vi "FaulhaberV3_Standalone.vi"() -> ()   [LabVIEW 2011]
panel:
  in  "1:x":i32(slide)=700 scale=-250000.0..250000.0
  in  "Tab Control":enum32{"command", "Script"}(tab)
  in  "commands":string[](array[string])=["Controlword?", "Modes of operation?", "Statusword?", "Position Actual Value?", "Controlword=0xF", "Modes of operation=1", "TargetPosition=-12345", "Controlword=0xF", "Controlword=0x1F", "Homing Method=37", "Modes of operation=6", "HomeOffset=23456", "Profile velocity?", "Profile velocity=1000", "Profile acceleration?", "Profile deceleration?", "Torque control parameters_Gain Kpi?", "Device data_Device nominal current?", "Device temperature_Winding temperature?", "Actual values_Motor current Id actual value?", "Current actual value?", "Motion profile type?", "Device Status?", "", "", "", "", ""]
  in  "Run":bool[](array[boolean])=[FALSE, FALSE, FALSE, FALSE, FALSE, FALSE, FALSE, FALSE, FALSE, FALSE, FALSE, FALSE, FALSE, FALSE, FALSE, FALSE, FALSE, FALSE, FALSE, FALSE, FALSE, FALSE, FALSE]
  out "return name":string="5000\r\n"
  out "return":i32
  out "Binary":bool[](array[boolean])
  out "Cluster 2":T1={"command"="goto abs", "Numeric"=0.0, "wait ms"=1000, "expected ssi"=235298.717399, "String"="go to low"}
  in  "start":bool
  out "Waveform Chart":dbl(graph)=2342.2826010000135
  in  "Timeout ms":i32=-1
  in  "Export ascii":bool
  in  "read ascii":bool
  in  "Next#":i32=259
  in  "List":T2(array[cluster])=[{"command"="LA", "Numeric"=30000.0, "wait ms"=10, "expected ssi"=0.0, "String"=""}, {"command"="M", "Numeric"=nan, "wait ms"=1000, "expected ssi"=0.0, "String"=""}, {"command"="LA", "Numeric"=0.0, "wait ms"=10, "expected ssi"=0.0, "String"=""}, {"command"="M", "Numeric"=nan, "wait ms"=1000, "expected ssi"=0.0, "String"=""}, {"command"="LA", "Numeric"=-30000.0, "wait ms"=10, "expected ssi"=0.0, "String"=""}, {"command"="M", "Numeric"=nan, "wait ms"=1000, "expected ssi"=0.0, "String"=""}, {"command"="LA", "Numeric"=0.0, "wait ms"=10, "expected ssi"=0.0, "String"=""}, {"command"="M", "Numeric"=nan, "wait ms"=1000, "expected ssi"=0.0, "String"=""}]
  in  "allowed ssi error":dbl=2000.0
  out "ssi in range":bool
  out "connect OK":bool
  out "error out":errorcluster
  in  "stop":bool
  in  "Axis # (nur1)":i16=1
  in  "Port, enter before start":refnum<visa-resource-name>="COM10"
  # "christianb:com10,D:com8"
  # "60000=10mm"
  # "closes comport\notherwise use STOP"
  # "Status ro\n0  ready on\n1 On\n2 Enabled\n3 Fault\n4 volt enabled\n5 quickstop\n6 on disabled\n7 Warning\n8 \n9 \n10 reached\n11 internal limit\n12  new point acept\n 13 follow error"
  # "Control\n0 on\n1 enable\n2 quick stop\n3 enable\n4 take set\n5 take immediately\n6 is relative\n7 faultreset\n8 halt\n9 no stop \n10 reached\n11\n12 point Acq"
  # "Einschalten\nControlword=0xF   Bit0,1,2,3, vorher 0x6?\nModes of operation=1 (PP)\n\nFahren\nTargetPosition=1234\nControlword=0xF könnte auch vorher sein\nControlword=0x1F  bit4 setzen, steigend=go, oder 3F sofort\n\nHoming method=37\nModes of operation=6 (Homing)\nHomeOffset=2345\nControlword=0x1F  bit 4 setzen\n?"
  # "software limits: \nPosition range limit_Min position range limit\nPosition range limit_Max position range limit\nSoftware position limit_Min position limit\nGNL, GPL\nSet LL<0, LL>0\nTEM Temperatur\nLPC 500  (mA)"
  # "Abfragen:\nPosition Actual Value?\nGAC\nGSP\nGRC  aktuelleer Strom\nG..."
  # "Parameter\nAC 5000\nDEC 5000\nSP 3000 (RPM=25mm/s)"
  # "-1 = stop\n>=0 restart"
  # "NaN expectet will not be checked"
  # "verlorener schritt=256*4 ysteps\nhalber ~200ssi (400 z)"
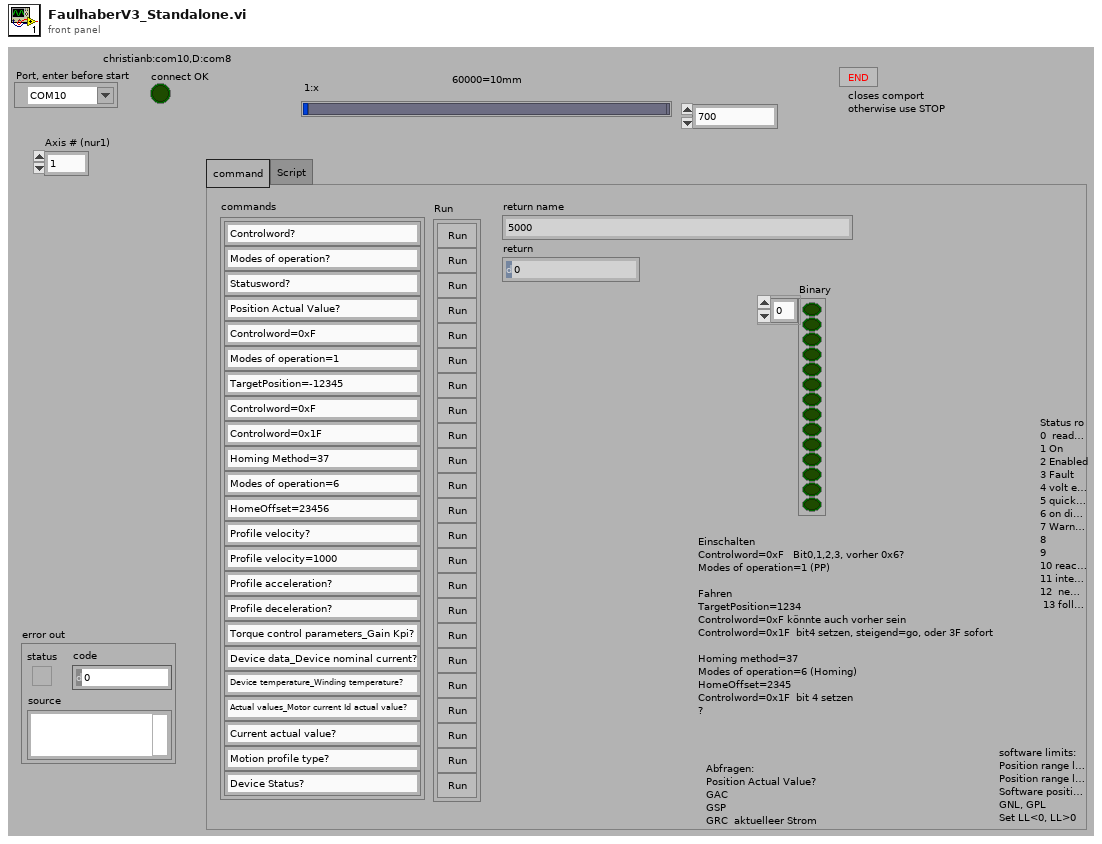
[diagram p1: front panel]
types:
  T1 = cluster{"command":string, "Numeric":dbl, "wait ms":i32, "expected ssi":dbl, "String":string}
  T2 = cluster{"command":string, "Numeric":dbl, "wait ms":i32, "expected ssi":dbl, "String":string}[]
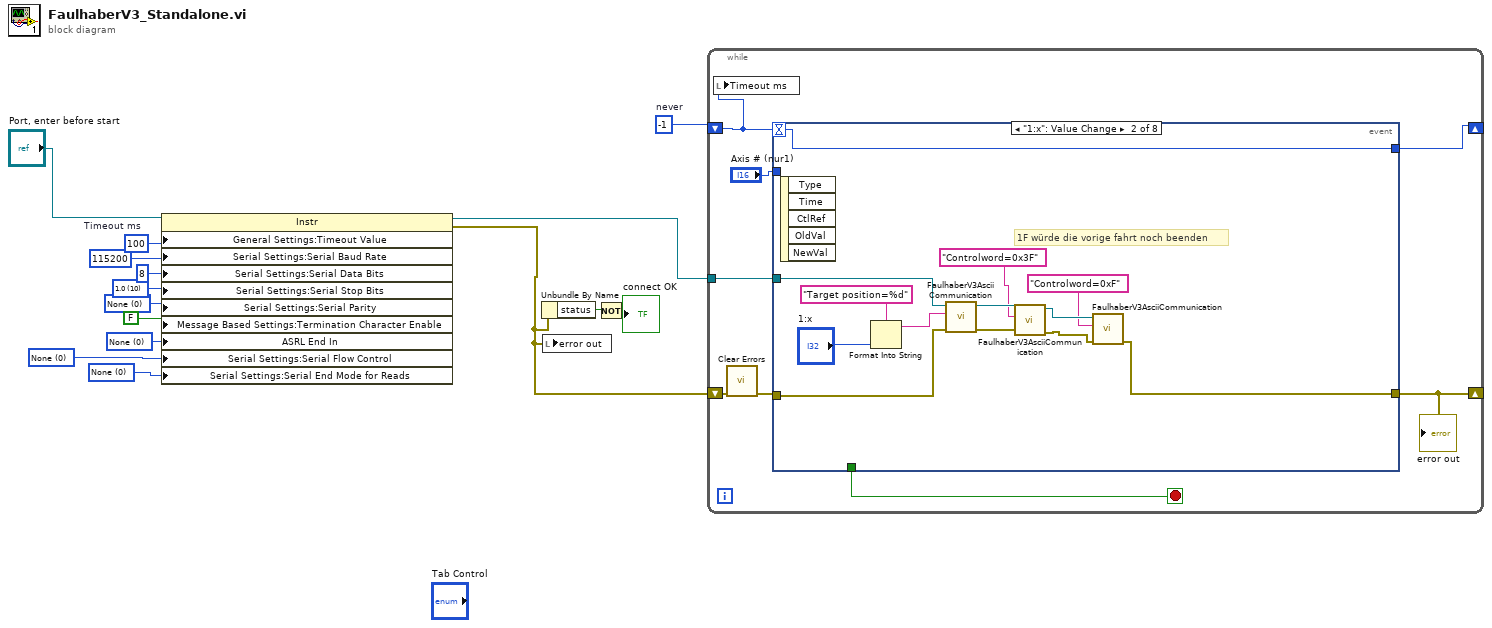
[diagram p0: block diagram]
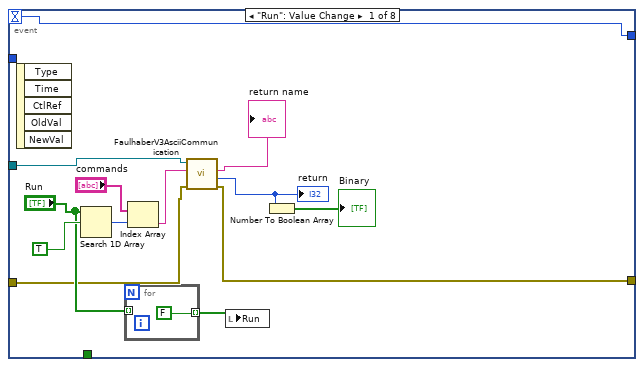
[diagram p2: hidden frame]
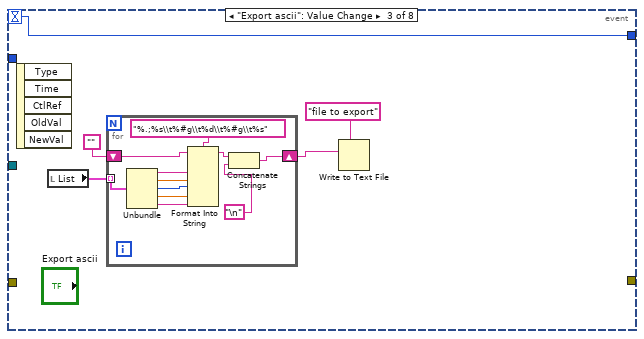
[diagram p3: hidden frame]
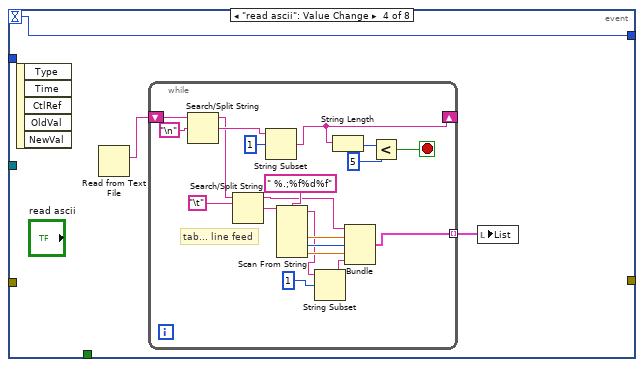
[diagram p4: hidden frame]
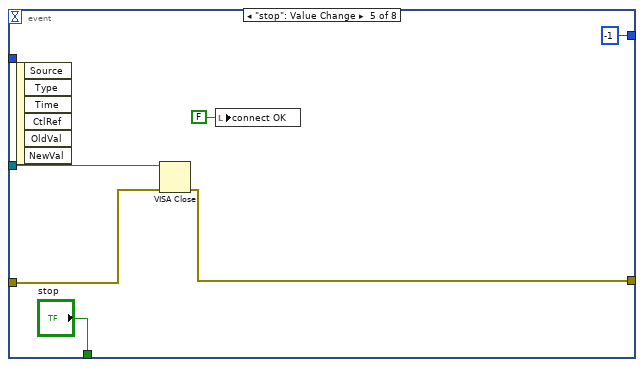
[diagram p5: hidden frame]
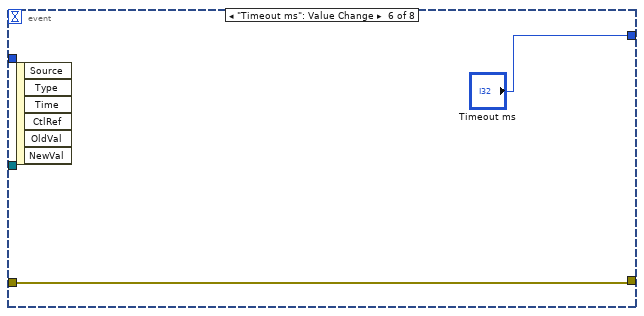
[diagram p6: hidden frame]
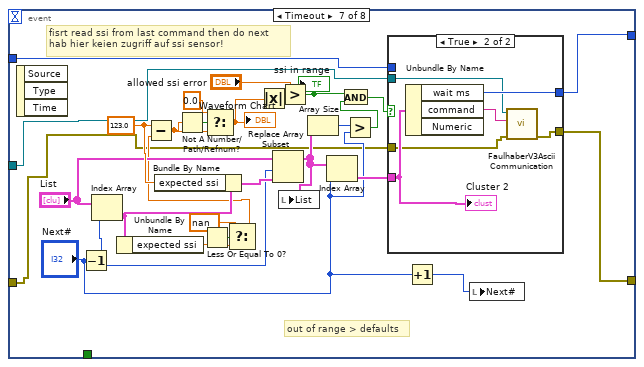
[diagram p7: hidden frame]
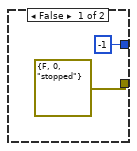
[diagram p8: hidden frame]
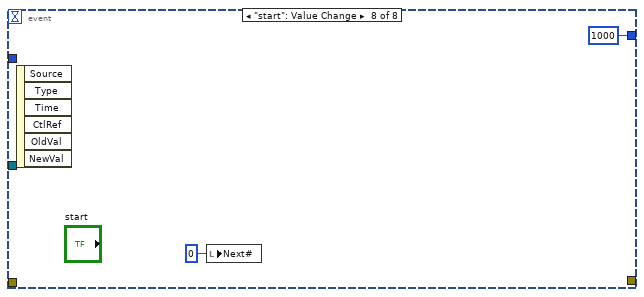
[diagram p9: hidden frame]
diagram:
  w2 = u16 0 items=["None", "Last Bit", "TermChar"] ("Serial Settings:End Mode for Reads")
  w7 = u32 100  # Timeout ms
  w9 = u16 10 items=["1.0"=10, "1.5"=15, "2.0"=20] ("Serial Settings:Stop Bits")
  w10 = u16 0 items=["None", "Odd", "Even", "Mark", "Space"] ("Serial Settings:Parity")
  w11 = u16 0 items=["None", "Last Bit", "TermChar"] ("Serial Settings:End Mode for Reads")
  w3 = u16 0 items=["None", "XON/XOFF", "RTS/CTS", "XON/XOFF & RTS/CTS", "DTR/DSR", "XON/XOFF & DTR/DSR"] ("Serial Settings:Flow Control")
  w13 = -1  # never
  n1 = property class="Instr"(reference="Port, enter before start", "General Settings:Timeout Value"=w7, "Serial Settings:Serial Baud Rate"=u32 115200 ("Serial Settings:Baud Rate"), "Serial Settings:Serial Data Bits"=u16 8 ("Serial Settings:Data Bits"), "Serial Settings:Serial Stop Bits"=w9, "Serial Settings:Serial Parity"=w10, "Message Based Settings:Termination Character Enable"=FALSE, "ASRL End In"=w2, "Serial Settings:Serial Flow Control"=w3, "Serial Settings:Serial End Mode for Reads"=w11) -> (reference out=w4:refnum<visa-resource-name>, error out=w1:errorcluster)  [unwired: 1 in]
  n2 = Unbundle By Name(w1) -> ("status"=w15:bool)
  n3 = local write "error out"(w1) -> ()
  n4 = Not(x=w15) -> (.not. x?=→"connect OK":bool)
  n5 = while {
    shift-right: [w22] -> _
    shift-left: w1 -> [w21]
    tunnel: w4 -> [w20]
    shift-right: [w16] -> _
    shift-left: w13 -> [w17]
    stop <- w23 stop-if-true
    n6 = local write "Timeout ms"(w17) -> ()
    n7 = call <vilib>:"Clear Errors.vi"("error in (no error)"=w21) -> ("error out"=w19:errorcluster)  [unwired: 6 out]
    n8 = event shown="[1] \"1:x\": Value Change" {
      selector: _ -> [_ _ _ _ _ _ _ _]
      dyn-events: _ -> [_ _ _ _ _ _ _ _]
      timeout: w17 -> [w30 w50 w51 w67 _ _ _ _]
      tunnel: [_ _ _ _ "stop" _ _ _] -> w23
      tunnel: [w27 w40 _ _ w93 w96 w115 _] -> w22
      tunnel: w19 -> [w29 w48 _ _ w94 w96 w98 _]
      tunnel: w20 -> [w28 w49 _ _ w92 _ w99 _]
      tunnel: "Axis # (nur1)" -> [_ _ _ _ _ _ w118 _]
      tunnel: [w30 w50 w51 w67 -1 ("wait ms") "Timeout ms" w116 1000 ("wait ms")] -> w16
      event "Run": Value Change {
        n9 = event-data() -> ()  [unwired: 6 out]
        n10 = Search 1D Array(1D array="Run", element=TRUE) -> (index of element=w34:i32)  [unwired: 1 out]
        n11 = for {
          tunnel: "Run" -> [_] mode=indexing
          tunnel: [FALSE ("element")] -> w31 mode=indexing
        }
        n12 = Index Array(array="commands", index=w34) -> (element=w25:string)
        n13 = call "FaulhaberV3AsciiCommunication.vi"("error in (no error)"=w29, "Befehl"=w25, "VISA resource name"=w28) -> ("error out"=w27:errorcluster, "returnValue"=w24:i32, "return"=→"return name":string)  [unwired: 5 in, 1 out]
        "return" <- w24
        n14 = local write "Run"(w31) -> ()
        n15 = Number To Boolean Array(number=w24) -> (Boolean array=→"Binary":bool[])
      }
      event "1:x": Value Change {
        # "1F würde die vorige fahrt noch beenden"
        n16 = event-data() -> ()  [unwired: 6 out]
        n17 = Format Into String(format string="Target position=%d", "1:x") -> (resulting string=w43:string)  [unwired: 2 in, 1 out]
        n18 = call "FaulhaberV3AsciiCommunication.vi"("error in (no error)"=w48, "Befehl"=w43, "VISA resource name"=w49) -> ("error out"=w46:errorcluster, "VISA resource name out"=w47:refnum<visa-resource-name>)  [unwired: 5 in, 2 out]
        n19 = call "FaulhaberV3AsciiCommunication.vi"("error in (no error)"=w46, "Befehl"="Controlword=0x3F" ("command"), "VISA resource name"=w47) -> ("error out"=w41:errorcluster, "VISA resource name out"=w39:refnum<visa-resource-name>)  [unwired: 5 in, 2 out]
        n20 = call "FaulhaberV3AsciiCommunication.vi"("error in (no error)"=w41, "Befehl"="Controlword=0xF" ("command"), "VISA resource name"=w39) -> ("error out"=w40:errorcluster)  [unwired: 5 in, 3 out]
      }
      event "Export ascii": Value Change {
        n21 = event-data() -> ()  [unwired: 6 out]
        n22 = local read "List"() -> (w55:T2)
        n23 = for {
          tunnel: w55 -> [w66] mode=indexing
          shift-right: [w58] -> w53
          shift-left: "" -> [w65]
          n24 = Unbundle(w66) -> ("command"=w64:string, "Numeric"=w63:dbl, "wait ms"=w62:i32, "expected ssi"=w61:dbl, "String"=w60:string)
          n25 = Format Into String(format string="%.;%s\\t%#g\\t%d\\t%#g\\t%s", initial string=w65, w64, w63, w62, w61, w60) -> (resulting string=w59:string)  [unwired: 1 in, 1 out]
          n26 = Concatenate Strings(w59, "\n") -> (w58:string)
        }
        n27 = Write to Text File(prompt (Choose or enter file path)="file to export", text=w53) -> ()  [unwired: 2 in, 3 out]
      }
      event "read ascii": Value Change {
        n28 = event-data() -> ()  [unwired: 6 out]
        n29 = Read from Text File() -> (text=w69:string)  [unwired: 4 in, 3 out]
        n30 = while {
          shift-right: [w76] -> _
          shift-left: w69 -> [w89]
          tunnel: [w84] -> w68 mode=indexing
          stop <- w73 stop-if-true
          # "tab... line feed"
          n31 = Search/Split String(string=w89, search string/char (-)="\n") -> (substring before match=w78:string, match + rest of string=w82:string)  [unwired: 1 in, 1 out]
          n32 = Search/Split String(string=w78, search string/char (-)="\t") -> (substring before match=w79:string, match + rest of string=w77:string)  [unwired: 1 in, 1 out]
          n33 = String Subset(string=w82, offset (0)=1) -> (substring=w76:string)  [unwired: 1 in]
          n34 = Scan From String(format string=" %.;%f%d%f", input string=w77) -> (remaining string=w71:string, output 1=w87:dbl, output 2=w86:i32, output 3=w85:dbl)  [unwired: 5 in, 2 out]
          n35 = String Subset(string=w71, offset (0)=1) -> (substring=w70:string)  [unwired: 1 in]
          n36 = String Length(string=w76) -> (length=w75:i32)
          n37 = Bundle(w79, w87, w86, w85, w70) -> (w84:cluster{string, dbl, i32, dbl, string})  [unwired: 1 in]
          n38 = Less?(x=w75, y=5) -> (x < y?=w73:bool)
        }
        n39 = local write "List"(w68) -> ()
      }
      event "stop": Value Change {
        n40 = event-data() -> ()  [unwired: 7 out]
        n41 = VISA Close(VISA resource name=w92, error in (no error)=w94) -> (error out=w93:errorcluster)
        n42 = local write "connect OK"(FALSE ("connect OK")) -> ()
      }
      event "Timeout ms": Value Change {
        n43 = event-data() -> ()  [unwired: 7 out]
      }
      event Timeout {
        w122 = 123.0 ("x")
        # "out of range > defaults"
        # "fisrt read ssi from last command then do next\nhab hier keien zugriff auf ssi sensor!"
        n44 = event-data() -> ()  [unwired: 4 out]
        n45 = Decrement(x="Next#") -> (x-1=w119:i32)
        n46 = Index Array(array="List", index=w119) -> (element=w123:T1)
        n47 = Unbundle By Name(w123) -> ("expected ssi"=w104:dbl)
        n48 = Bundle By Name(cluster=w123, "expected ssi"=w122) -> (w120:T1)
        n49 = Less Or Equal To 0?(x=w104) -> (x <= 0?=w105:bool)
        n50 = Select(t=nan, s=w105, f=w104) -> (s? t:f=w103:dbl)
        n51 = Subtract(x=w122, y=w103) -> (x-y=w107:dbl)
        n52 = Not A Number/Path/Refnum?(number/path/refnum=w107) -> (NaN/Path/Refnum?=w108:bool)
        n53 = Select(t=0.0, s=w108, f=w107) -> (s? t:f=w106:dbl)
        "Waveform Chart" <- w106
        n54 = Absolute Value(x=w106) -> (abs(x)=w125:dbl)
        n55 = Replace Array Subset(array="List", new element=w120, index=w119) -> (w114:T2)
        n56 = local write "List"(w114) -> ()
        n57 = Greater?(x="allowed ssi error", y=w125) -> (0:w111:bool)
        "ssi in range" <- w111
        n58 = Array Size(array=w114) -> (size(s)=w113:i32)
        n59 = Index Array(array=w114, index="Next#") -> (element=w117:T1)
        n60 = Greater?(x=w113, y="Next#") -> (0:w112:bool)
        n61 = And(x=w111, y=w112) -> (x .and. y?=w110:bool)
        n62 = case shown="True" w110 {
          tunnel: w118 -> [_ _]
          tunnel: w99 -> [_ w129]
          tunnel: w117 -> [_ w132]
          tunnel: w98 -> [_ w130]
          tunnel: [-1 ("wait ms") w133] -> w116
          tunnel: [errorcluster {"status"=FALSE, "code"=0, "source"="stopped"} ("error out") w131] -> w115
          frame False {
          }
          frame True {
            n63 = Unbundle By Name(w132) -> ("wait ms"=w133:i32, "command"=w128:string)  [unwired: 1 out]
            n64 = call "FaulhaberV3AsciiCommunication.vi"("error in (no error)"=w130, "Befehl"=w128, "VISA resource name"=w129) -> ("error out"=w131:errorcluster)  [unwired: 5 in, 3 out]
            "Cluster 2" <- w132
          }
        }
        n65 = Increment(x="Next#") -> (x+1=w100:i32)
        n66 = local write "Next#"(w100) -> ()
      }
      event "start": Value Change {
        n67 = event-data() -> ()  [unwired: 7 out]
        n68 = local write "Next#"(0 ("Next#")) -> ()
      }
    }
    "error out" <- w22
  }
